vi "创建图像缓存.vi"() -> (3 "簇":T2)   [LabVIEW 2015]
uses:
  <vilib>/vision/Image Controls.llb/IMAQ Image.ctl
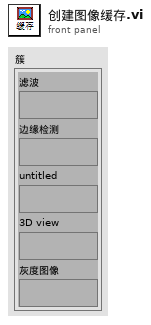
[diagram p1: front panel]
types:
  T1 = typedef "IMAQ Image.ctl" = refnum<image>
  T2 = cluster{"滤波":T1, "边缘检测":T1, "untitled":T1, "3D view":T1, "灰度图像":T1}
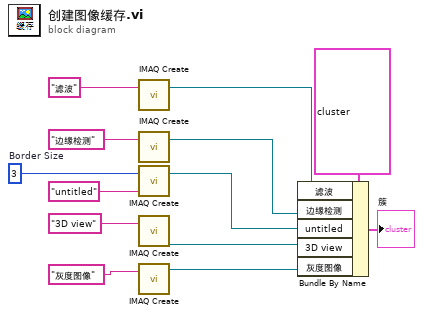
[diagram p0: block diagram]
diagram:
  w6 = 3  # Border Size
  n1 = call "IMAQ Create"("Image Name"="滤波") -> ("New Image"=w8:T1)  [unwired: 4 in, 1 out]
  n2 = call "IMAQ Create"("Image Name"="边缘检测") -> ("New Image"=w9:T1)  [unwired: 4 in, 1 out]
  n3 = call "IMAQ Create"("Border Size"=w6, "Image Name"="untitled") -> ("New Image"=w10:T1)  [unwired: 2 in, 2 out]
  n4 = call "IMAQ Create"("Image Name"="3D view") -> ("New Image"=w11:T1)  [unwired: 4 in, 1 out]
  n5 = call "IMAQ Create"("Image Name"="灰度图像") -> ("New Image"=w12:T1)  [unwired: 4 in, 1 out]
  n6 = Bundle By Name(cluster=T2 {"滤波"=refnum, "边缘检测"=refnum, "untitled"=refnum, "3D view"=refnum, "灰度图像"=refnum}, "滤波"=w8, "边缘检测"=w9, "untitled"=w10, "3D view"=w11, "灰度图像"=w12) -> (→"簇":T2)
